vi "Training ML Model.vi"() -> ()   [LabVIEW 2018]
uses:
  <vilib>/addons/AML/Classification/SVM/Controls/aml_SVM Parameters.ctl
  <vilib>/addons/AML/Classification/SVM/Controls/aml_SVM Type.ctl
  <vilib>/addons/AML/Classification/SVM/Controls/aml_SVM Kernel Settings.ctl
  <vilib>/addons/AML/Classification/SVM/Controls/aml_SVM Kernel Type.ctl
  <vilib>/addons/AML/Classification/Common/Controls/aml_Cross Validation Configuration.ctl
  <vilib>/addons/AML/Classification/Common/Controls/aml_Evaluation Configuration.ctl
  <vilib>/addons/AML/Classification/Common/Controls/aml_Metric Average.ctl
  <vilib>/addons/AML/Classification/SVM/Classes/AML SVM.lvclass
  C:/Program Files (x86)/National Instruments/LabVIEW 2018/vi.lib/addons/AML/Classification/Common/Classes/AML Classification.lvclass
  <vilib>/addons/AML/Data/Load Training Data (2D Array).vi
  <vilib>/addons/AML/Feature Manipulation/Normalize (One Shot).vi
  <vilib>/addons/AML/Classification/Initialize Classification Model (SVM, Set).vi
  <vilib>/addons/AML/Analytics and Machine Learning.lvlib
  <vilib>/gmath/NI_Gmath.lvlib
panel:
  out "Feature col":string[](array[string])
  out "Feature row":string[](array[string])
  out "Correlation matrix":dbl[][](array[numeric])
  out "error out":errorcluster
  in  "Tab Control":T1(tab)
  in  "Chhose training data file (CSV)":path
  out "feature trend":dbl[][](graph)
  in  "Choose the directory where you want to save your ML model":path
  out "metrics (cross validation)":T2
  in  "coef0":dbl
  in  "gamma":dbl=0.5
  in  "degree":i32=3
  in  "nu":dbl=0.5
  in  "c":dbl=1.0
  in  "kernel type":enum32{"Linear", "Polynomial", "RBF", "Sigmoid"}(ring)
  in  "SVM type":enum32{"C_SVC", "NU_SVC"}(ring)
  out "Correlation Matrix Heatmap":dbl[][](graph)
  # "Correlation Matrix"
  # "SVM"
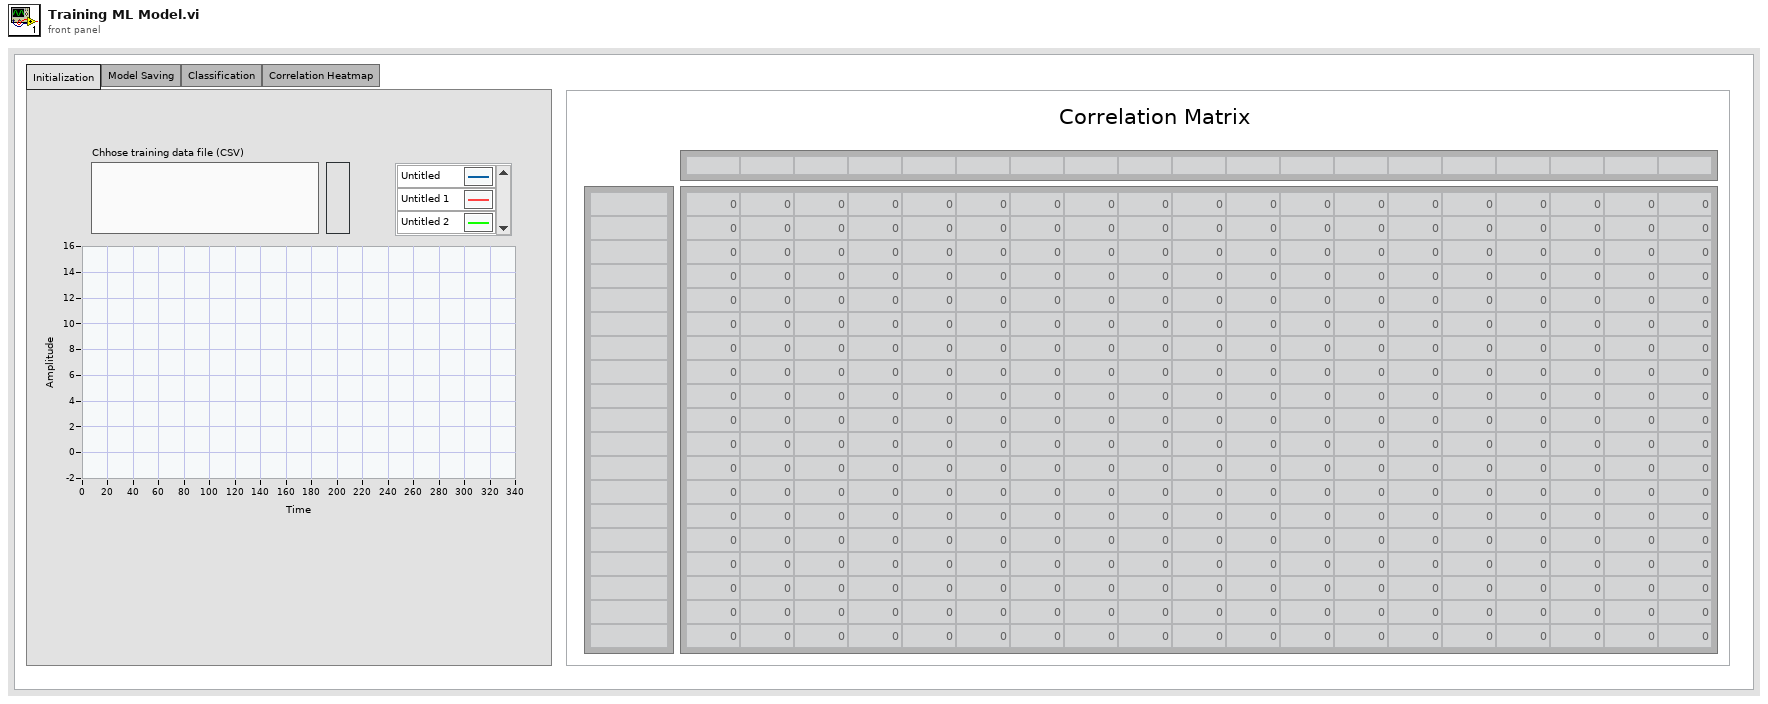
[diagram p1: front panel]
types:
  T1 = enum32{"Initialization", "Model Saving", "Classification", "Correlation Heatmap"}
  T2 = cluster{"accuracy":dbl, "precision":dbl, "recall":dbl, "f1 score":dbl}
  T3 = cluster{"with label column?":bool, "label column index":i32}
  T4 = typedef "Analytics and Machine Learning.lvlib/aml_Cross Validation Configuration.ctl" = cluster{"enable?":bool, "number of folds":u32, "metric configuration":T5}
  T5 = typedef "Analytics and Machine Learning.lvlib/aml_Evaluation Configuration.ctl" = cluster{"average method":T6, "positive label":i32}
  T6 = typedef "Analytics and Machine Learning.lvlib/aml_Metric Average.ctl" = enum16{"Micro", "Macro", "Weighted", "Binary"}
  T7 = typedef "Analytics and Machine Learning.lvlib/aml_SVM Parameters.ctl" = cluster{"SVM type":T8, "c":dbl, "nu":dbl, "kernel settings":T9, "weighted c":cluster{"label":i32, "weight":dbl}[], "tolerance":dbl, "max iteration":i32}
  T8 = typedef "Analytics and Machine Learning.lvlib/aml_SVM Type.ctl" = enum32{"C_SVC", "NU_SVC"}
  T9 = typedef "Analytics and Machine Learning.lvlib/aml_SVM Kernel Settings.ctl" = cluster{"type":T10, "degree":i32, "gamma":dbl, "coef0":dbl}
  T10 = typedef "Analytics and Machine Learning.lvlib/aml_SVM Kernel Type.ctl" = enum32{"Linear", "Polynomial", "RBF", "Sigmoid"}
  T11 = enum16{"open", "replace", "create", "open or create", "replace or create", "replace or create with confirmation"}
  T12 = typedef "Analytics and Machine Learning.lvlib/aml_Model Metrics.ctl" = cluster{"accuracy":dbl, "precision":dbl, "recall":dbl, "f1 score":dbl}
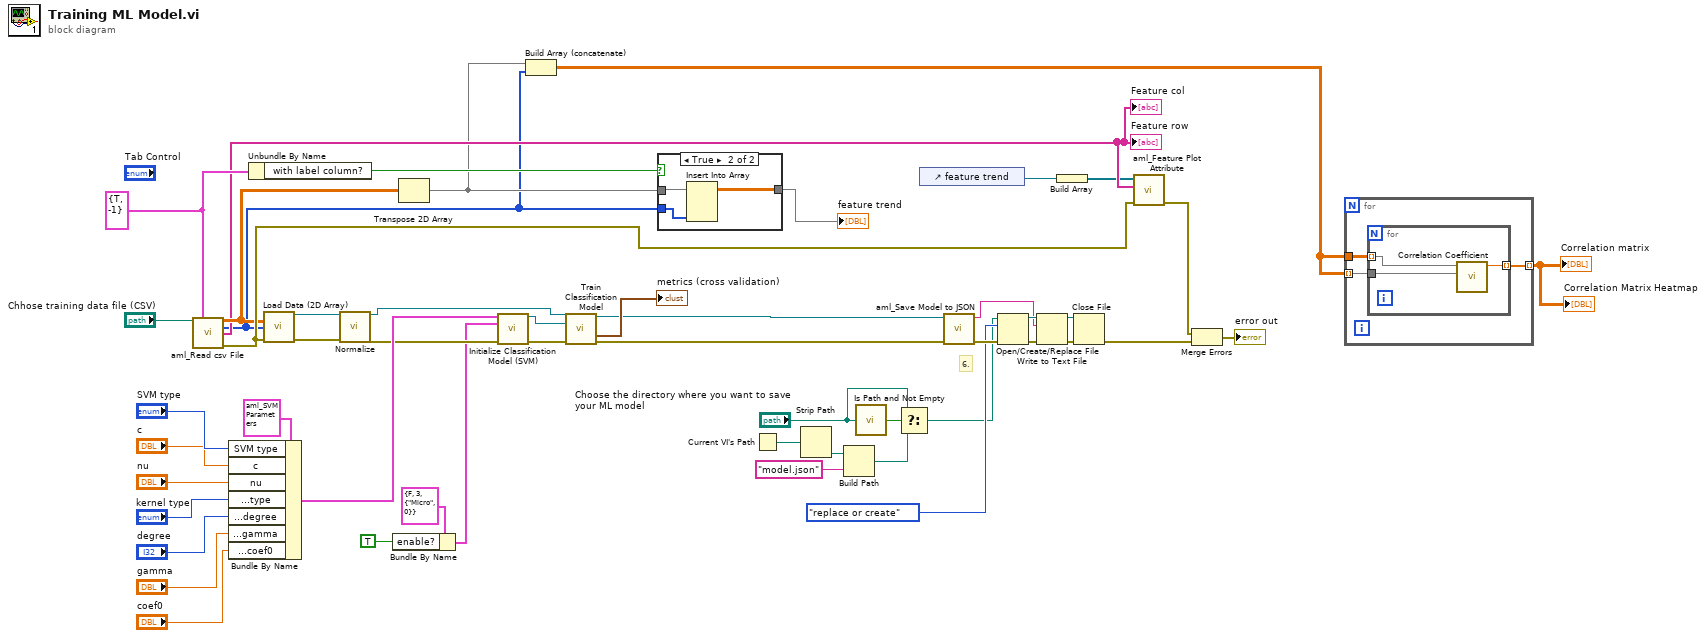
[diagram p0: block diagram]
diagram:
  w15 = T3 {"with label column?"=TRUE, "label column index"=-1} ("label settings")
  # "6."
  n1 = call <vilib>:"aml_Read csv File.vi"("csv file path"="Chhose training data file (CSV)", "label setting"=w15) -> ("data"=w9:dbl[][], "data label"=w5:i32[], "feature names"=w7:string[], "error out"=w50:errorcluster)  [unwired: 10 in]
  "Feature row" <- w7
  "Feature col" <- w7
  n2 = Bundle By Name(cluster=T7 {"SVM type"=enum."C_SVC", "c"=1.0, "nu"=0.5, "kernel settings"={"type"=enum."Linear", "degree"=3, "gamma"=0.5, "coef0"=0.0}, "weighted c"=[], "tolerance"=0.001, "max iteration"=100000} ("hyperparameters"), "SVM type"="SVM type", "c"="c", "nu"="nu", "kernel settings.type"="kernel type", "kernel settings.degree"="degree", "kernel settings.gamma"="gamma", "kernel settings.coef0"="coef0") -> (w24:T7)
  n3 = Unbundle By Name(w15) -> ("with label column?"=w14:bool)
  n4 = call-poly <vilib>:"Load Data (2D Array).vi"("data"=w9, "data labels"=w5, "error in (no error)"=w50) -> ("model out"=w48:refnum<class "AML Analytics Model.lvclass">, "error out"=w47:errorcluster)  [unwired: 11 in]
  n5 = call-poly <vilib>:"Normalize.vi"("model in"=w48, "error in (no error)"=w47) -> ("model out"=w17:refnum<class "AML Analytics Model.lvclass">, "error out"=w19:errorcluster)  [unwired: 11 in, 1 out]
  n6 = Bundle By Name(cluster=T4 {"enable?"=FALSE, "number of folds"=3, "metric configuration"={"average method"=enum."Micro", "positive label"=0}} ("cross validation configuration"), "enable?"=TRUE) -> (w18:T4)
  n7 = Transpose 2D Array(2D array=w9) -> (transposed array=w6:dbl[][])
  n8 = call-poly <vilib>:"Initialize Classification Model (SVM).vi"("hyperparameters"=w24, "cross validation configuration"=w18, "error in (no error)"=w19) -> ("untrained SVM Model"=w22:refnum<class "AML SVM.lvclass">, "error out"=w23:errorcluster)  [unwired: 11 in]
  n9 = Build Array (concatenate)(w6, w5) -> (w4:dbl[][])
  n10 = call <vilib>:"Train Classification Model.vi"("model in"=w17, "classification model info in"=w22, "error in (no error)"=w23) -> ("model out"=w13:refnum<class "AML Analytics Model.lvclass">, "metrics"=→"metrics (cross validation)":T12, "error out"=w10:errorcluster)  [unwired: 8 in, 2 out]
  n11 = case shown="True" w14 {
    tunnel: w5 -> [_ w54]
    tunnel: w6 -> [w52 w55]
    tunnel: [w52 w53] -> w3
    frame False {
    }
    frame True {
      n12 = Insert Into Array(array=w55, new element=w54) -> (w53:dbl[][])  [unwired: 2 in]
    }
  }
  "feature trend" <- w3
  n13 = Current VI's Path() -> (path=w42:path)
  n14 = Strip Path(path=w42) -> (stripped path=w41:path)  [unwired: 1 out]
  n15 = Build Path(base path=w41, name or relative path="model.json") -> (appended path=w44:path)
  n16 = call <vilib>:"Is Path and Not Empty.vi"("path"="Choose the directory where you want to save your ML model") -> ("Is Path and Not Empty?"=w46:bool)  [unwired: 4 in]
  n17 = Select(t="Choose the directory where you want to save your ML model", s=w46, f=w44) -> (s? t:f=w36:path)
  n18 = control-ref of="feature trend"() -> (w2:refnum<vi>)
  n19 = call <vilib>:"aml_Save Model to JSON.vi"("error in (no error)"=w10, "model in"=w13) -> ("error out"=w38:errorcluster, "JSON string"=w33:string)  [unwired: 8 in]
  n20 = Open/Create/Replace File(file path (use dialog)=w36, error in=w38, operation (0:open)=T11."replace or create") -> (refnum out=w35:refnum<file>, error out=w39:errorcluster)  [unwired: 3 in, 1 out]
  n21 = Write to Text File(file (use dialog)=w35, text=w33, error in=w39) -> (refnum out=w34:refnum<file>, error out=w40:errorcluster)  [unwired: 1 in, 1 out]
  n22 = Build Array(w2) -> (w1:refnum<vi>[])
  n23 = Close File(refnum=w34, error in=w40) -> (error out=w51:errorcluster)  [unwired: 1 out]
  n24 = call <vilib>:"aml_Feature Plot Attribute.vi"("error in (no error)"=w50, "feature names"=w7, "appended array"=w1) -> ("error in (no error)"=w12:errorcluster)  [unwired: 8 in]
  n25 = Merge Errors(w12, w51) -> (→"error out":errorcluster)
  n26 = for {
    tunnel: w4 -> [w58] mode=indexing
    tunnel: w4 -> [w57]
    tunnel: [w56] -> w8 mode=indexing
    n27 = for {
      tunnel: w58 -> [w59]
      tunnel: w57 -> [w60] mode=indexing
      tunnel: [w61] -> w56 mode=indexing
      n28 = call <vilib>:"Correlation Coefficient.vi"("Y"=w59, "X"=w60) -> ("correlation coefficient r"=w61:dbl)  [unwired: 8 in, 1 out]
    }
  }
  "Correlation matrix" <- w8
  "Correlation Matrix Heatmap" <- w8
